vi "Update Fields Table for Spartan 5.1.vi"(8 "error in (no error)":errorcluster, 10 "Spartan Install Dir":path, 11 "Connection Refnum":T1) -> (0 "error out":errorcluster, 3 "Connection Refnum":T1)   [LabVIEW 2011]
uses:
  Summitek EXT/ODBC/SQL Controls/Connection Refnum.ctl
  Field Record.ctl
  Field DataTypes.ctl
  Field NextItem.ctl
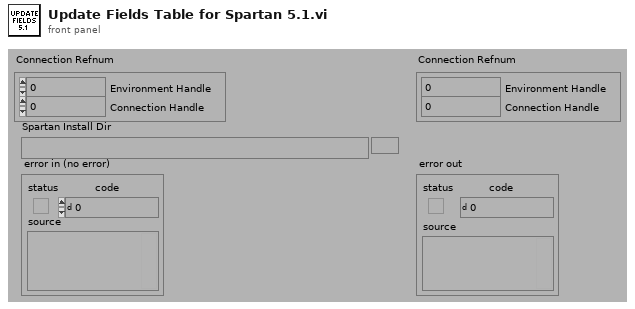
[diagram p1: front panel]
types:
  T1 = typedef "Connection Refnum.ctl" = cluster{"Environment Handle":i32, "Connection Handle":i32}
  T2 = typedef "Field Record.ctl" = cluster{"ixField":i32, "iSequenceOrder":i32, "sxFieldId":string, "sxSequenceId":string, "sDisplayName":string, "sValue":string, "sUnits":string, "nDataType":T3, "nNextItem":T4, "fSystem":bool, "fSystemValue":bool, "fRequired":bool, "fSetAtTest":bool, "fTestField":bool, "fDeleted":bool, "fIndexed":bool, "fFreeList":bool}
  T3 = typedef "Field DataTypes.ctl" = enum32{"text", "numeric", "list", "timestamp", "boolean"}
  T4 = typedef "Field NextItem.ctl" = enum32{"Reset", "Retain", "Auto-Increment"}
  T5 = enum16{"tdm_file", "tdm_channelgroup", "tdm_channel"}
  T6 = typedef "Statement Refnum.ctl" = cluster{"Statement Handle":i32, "Parameter Number":u16}
  T7 = typedef "DataFinder Indexed Property DataTypes.ctl" = enum32{"not optimized", "string", "double", "integer"}
  T8 = cluster{"DisplayName":string, "DataType":T7, "BuiltIn":bool}[]
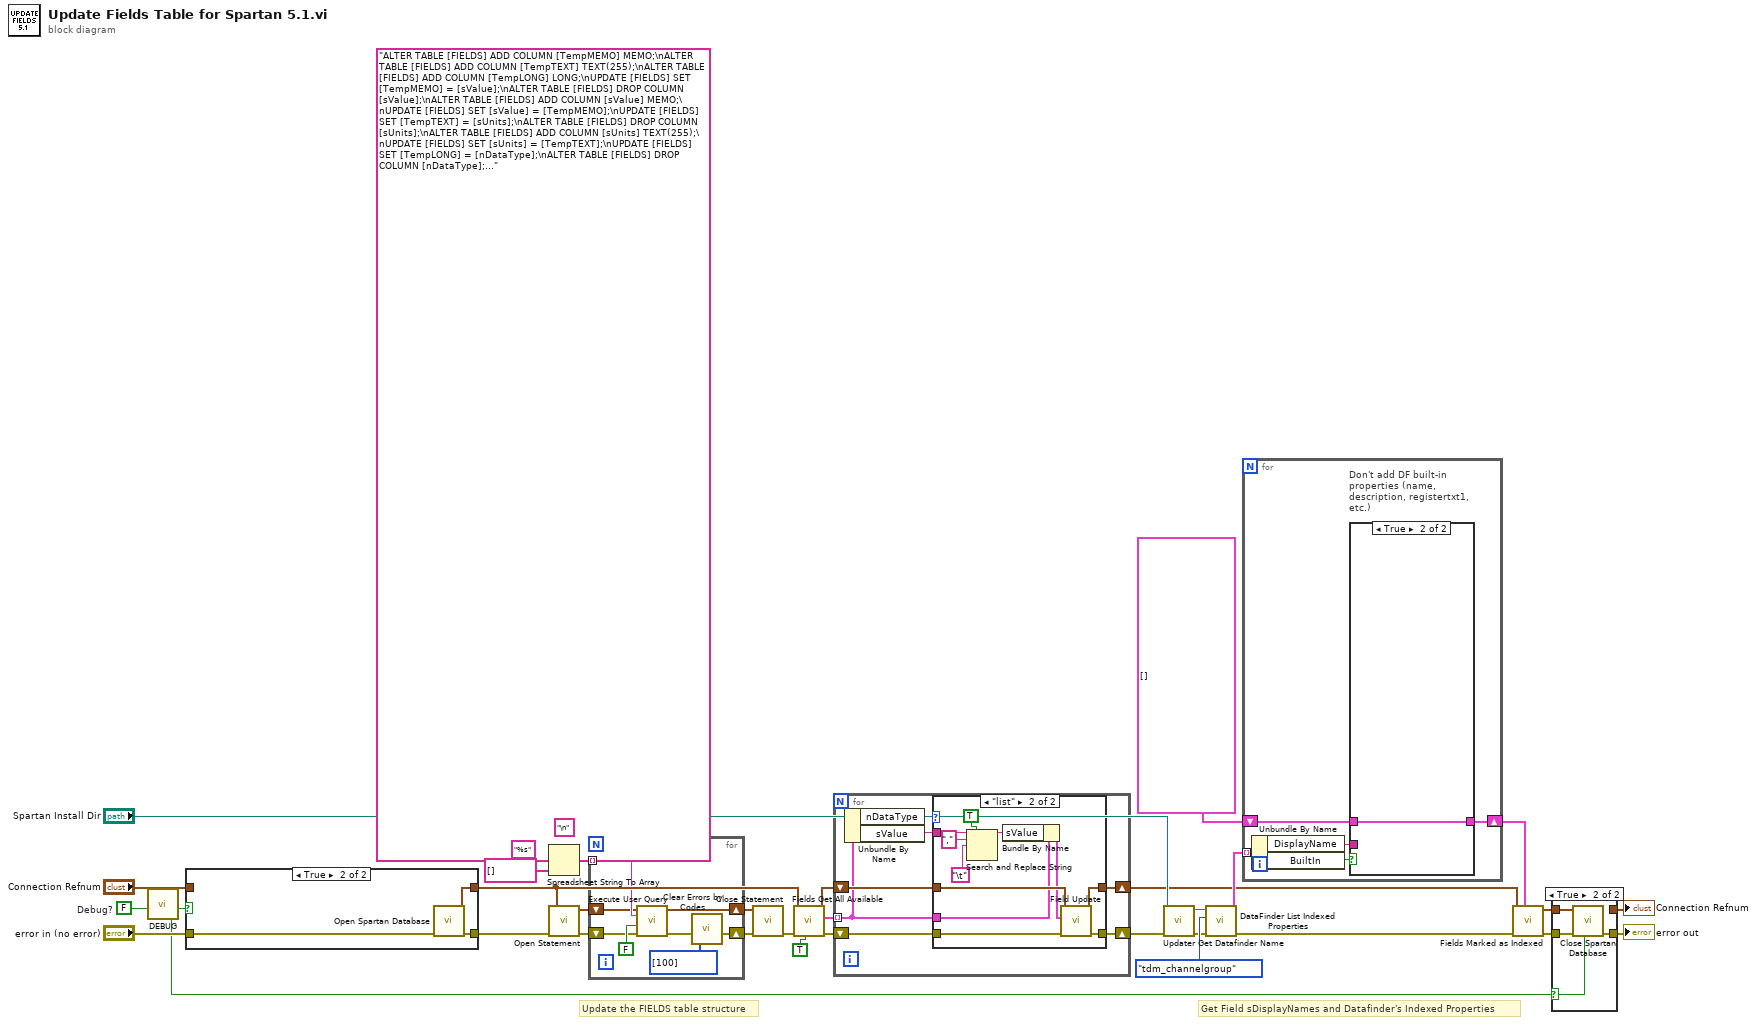
[diagram p0: block diagram]
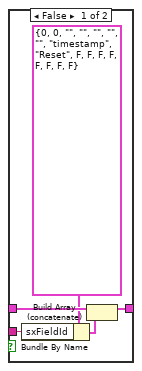
[diagram p5: hidden frame]
diagram:
  w1 = TRUE ("Combine All? (f)")
  w29 = FALSE  # Debug?
  # "Update the FIELDS table structure"
  # "Get Field sDisplayNames and Datafinder's Indexed Properties"
  n1 = call "DEBUG.vi"("Dev DEBUG? (f)"=w29) -> ("DEBUG?"=w24:bool)  [unwired: 1 in, 5 out]
  n2 = case shown="True" w24 {
    tunnel: "Connection Refnum" -> [w36 _]
    tunnel: "error in (no error)" -> [w35 w39]
    tunnel: [w35 w38] -> w9
    tunnel: [w36 w37] -> w7
    frame False {
    }
    frame True {
      n3 = call "Open Spartan Database.vi"("error in (no error)"=w39) -> ("error out"=w38:errorcluster, "Connection Refnum"=w37:T1)  [unwired: 2 in, 7 out]
    }
  }
  n4 = Spreadsheet String To Array(delimiter (Tab)="\n", format string="%s", spreadsheet string="ALTER TABLE [FIELDS] ADD COLUMN [TempMEMO] MEMO;\nALTER TABLE [FIELDS] ADD COLUMN [TempTEXT] TEXT(255);\nALTER TABLE [FIELDS] ADD COLUMN [TempLONG] LONG;\nUPDATE [FIELDS] SET [TempMEMO] = [sValue];\nALTER TABLE [FIELDS] DROP COLUMN [sValue];\nALTER TABLE [FIELDS] ADD COLUMN [sValue] MEMO;\nUPDATE [FIELDS] SET [sValue] = [TempMEMO];\nUPDATE [FIELDS] SET [TempTEXT] = [sUnits];\nALTER TABLE [FIELDS] DROP COLUMN [sUnits];\nALTER TABLE [FIELDS] ADD COLUMN [sUnits] TEXT(255);\nUPDATE [FIELDS] SET [sUnits] = [TempTEXT];\nUPDATE [FIELDS] SET [TempLONG] = [nDataType];\nALTER TABLE [FIELDS] DROP COLUMN [nDataType];\nALTER TABLE [FIELDS] ADD COLUMN [nDataType] LONG;\nUPDATE [FIELDS] SET [nDataType] = [TempLONG];\nUPDATE [FIELDS] SET [TempLONG] = [nNextItem];\nALTER TABLE [FIELDS] DROP COLUMN [nNextItem];\nALTER TABLE [FIELDS] ADD COLUMN [nNextItem] LONG;\nUPDATE [FIELDS] SET [nNextItem] = [TempLONG];\nUPDATE [FIELDS] SET [TempLONG] = [fSystem];\nALTER TABLE [FIELDS] DROP COLUMN [fSystem];\nALTER TABLE [FIELDS] ADD COLUMN [fSystem] LONG;\nUPDATE [FIELDS] SET [fSystem] = [TempLONG];\nUPDATE [FIELDS] SET [TempLONG] = [fSystemValue];\nALTER TABLE [FIELDS] DROP COLUMN [fSystemValue];\nALTER TABLE [FIELDS] ADD COLUMN [fSystemValue] LONG;\nUPDATE [FIELDS] SET [fSystemValue] = [TempLONG];\nUPDATE [FIELDS] SET [TempLONG] = [fRequired];\nALTER TABLE [FIELDS] DROP COLUMN [fRequired];\nALTER TABLE [FIELDS] ADD COLUMN [fRequired] LONG;\nUPDATE [FIELDS] SET [fRequired] = [TempLONG];\nUPDATE [FIELDS] SET [TempLONG] = [fSetAtTest];\nALTER TABLE [FIELDS] DROP COLUMN [fSetAtTest];\nALTER TABLE [FIELDS] ADD COLUMN [fSetAtTest] LONG;\nUPDATE [FIELDS] SET [fSetAtTest] = [TempLONG];\nUPDATE [FIELDS] SET [TempLONG] = [fTestField];\nALTER TABLE [FIELDS] DROP COLUMN [fTestField];\nALTER TABLE [FIELDS] ADD COLUMN [fTestField] LONG;\nUPDATE [FIELDS] SET [fTestField] = [TempLONG];\nUPDATE [FIELDS] SET [TempLONG] = [fDeleted];\nALTER TABLE [FIELDS] DROP COLUMN [fDeleted];\nALTER TABLE [FIELDS] ADD COLUMN [fDeleted] LONG;\nUPDATE [FIELDS] SET [fDeleted] = [TempLONG];\nUPDATE [FIELDS] SET [TempLONG] = [fIndexed];\nALTER TABLE [FIELDS] DROP COLUMN [fIndexed];\nALTER TABLE [FIELDS] ADD COLUMN [fIndexed] LONG;\nUPDATE [FIELDS] SET [fIndexed] = [TempLONG];\nUPDATE [FIELDS] SET [TempLONG] = [fFreeList];\nALTER TABLE [FIELDS] DROP COLUMN [fFreeList];\nALTER TABLE [FIELDS] ADD COLUMN [fFreeList] LONG;\nUPDATE [FIELDS] SET [fFreeList] = [TempLONG];\nALTER TABLE [FIELDS] DROP COLUMN [TempMEMO];\nALTER TABLE [FIELDS] DROP COLUMN [TempTEXT];\nALTER TABLE [FIELDS] DROP COLUMN [TempLONG];" ("User Query"), array type (2D Dbl)=string[] []) -> (array=w17:string[])
  n5 = call "Open Statement.vi"("error in (no error)"=w9, "Connection Refnum"=w7) -> ("error out"=w14:errorcluster, "Statement Refnum"=w13:T6)  [unwired: 4 out]
  n6 = for {
    shift-right: [w40] -> w12
    shift-left: w14 -> [w44]
    tunnel: w17 -> [w46] mode=indexing
    shift-right: [w43] -> w11
    shift-left: w13 -> [w45]
    n7 = call "Execute User Query.vi"("error in (no error)"=w44, "Return Data? (f)"=FALSE, "User Query"=w46, "Statement Refnum"=w45) -> ("error out"=w41:errorcluster, "Statement Refnum"=w43:T6)  [unwired: 2 out]
    n8 = call "Clear Errors by Codes.vi"("Error Codes\nto Clear (Empty)"=i32[] [100] ("Error Codes\nto Clear (Empty)"), "error in (no error)"=w41) -> ("error out"=w40:errorcluster)  [unwired: 5 out]
  }
  n9 = call "Close Statement.vi"("error in (no error)"=w12, "Statement Refnum"=w11) -> ("error out"=w8:errorcluster)  [unwired: 5 out]
  n10 = call "Fields Get All Available.vi"("Combine All? (f)"=w1, "Include Deleted? (F)"=w1, "error in (no error)"=w8, "Connection Refnum"=w7) -> ("error out"=w6:errorcluster, "System or ALL Combined Fields"=w2:T2[], "Connection Refnum"=w4:T1)  [unwired: 2 in, 3 out]
  n11 = for {
    shift-right: [w50] -> w5
    shift-left: w6 -> [w51]
    shift-right: [w49] -> w3
    shift-left: w4 -> [w52]
    tunnel: w2 -> [w48] mode=indexing
    n12 = Unbundle By Name(w48) -> ("nDataType"=w54:T3, "sValue"=w53:string)
    n13 = case shown="\"list\"" w54 {
      tunnel: w53 -> [_ w61]
      tunnel: w52 -> [w55 w66]
      tunnel: w51 -> [w56 w67]
      tunnel: [w56 w65] -> w50
      tunnel: [w55 w64] -> w49
      tunnel: w48 -> [_ w63]
      frame Default {
      }
      frame "list" {
        n14 = Search and Replace String(replace all?=TRUE ("replace all? (F)"), input string=w61, search string=",", replace string="\t") -> (result string=w59:string)  [unwired: 1 in, 6 out]
        n15 = Bundle By Name(cluster=w63, "sValue"=w59) -> (w62:T2)
        n16 = call "Field Update.vi"("error in (no error)"=w67, "Field Record"=w62, "Connection Refnum"=w66) -> ("error out"=w65:errorcluster, "Connection Refnum"=w64:T1)  [unwired: 7 out]
      }
    }
  }
  n17 = call "Updater Get Datafinder Name.vi"("error in (no error)"=w5, "spartan install dir"="Spartan Install Dir") -> ("error out"=w27:errorcluster, "datafinder name"=w26:string)  [unwired: 8 out]
  n18 = call "DataFinder List Indexed Properties.vi"("error in (no error)"=w27, "Type (tdm_file)"=T5."tdm_channelgroup", "DataFinder (\"My DataFinder\")"=w26) -> ("error out"=w22:errorcluster, "Indexed Properties"=w33:T8)  [unwired: 7 out]
  n19 = for {
    tunnel: w33 -> [w72] mode=indexing
    shift-right: [w68] -> w21
    shift-left: T2[] [] ("Fields In") -> [w69]
    n20 = Unbundle By Name(w72) -> ("DisplayName"=w71:string, "BuiltIn"=w70:bool)
    n21 = case "Don't add DF built-in\nproperties (name,\ndescription, registertxt1,\netc.)" shown="True" w70 {
      tunnel: w71 -> [w77 _]
      tunnel: w69 -> [w76 w78]
      tunnel: [w74 w78] -> w68
      frame False {
        n22 = Bundle By Name(cluster=T2 {"ixField"=0, "iSequenceOrder"=0, "sxFieldId"="", "sxSequenceId"="", "sDisplayName"="", "sValue"="", "sUnits"="", "nDataType"=enum."timestamp", "nNextItem"=enum."Reset", "fSystem"=FALSE, "fSystemValue"=FALSE, "fRequired"=FALSE, "fSetAtTest"=FALSE, "fTestField"=FALSE, "fDeleted"=FALSE, "fIndexed"=FALSE, "fFreeList"=FALSE} ("Field Record"), "sxFieldId"=w77) -> (w75:T2)
        n23 = Build Array (concatenate)(w76, w75) -> (w74:T2[])
      }
      frame True {
      }
    }
  }
  n24 = call "Fields Marked as Indexed.vi"("Fields In"=w21, "error in (no error)"=w22, "Connection Refnum"=w3) -> ("error out"=w19:errorcluster, "Connection Refnum"=w20:T1)  [unwired: 7 out]
  n25 = case shown="True" w24 {
    selector: w24 -> [_ w81]
    tunnel: w19 -> [w80 w84]
    tunnel: [w79 _] -> w28
    tunnel: [w80 w83] -> w30
    tunnel: w20 -> [w79 w82]
    frame False {
    }
    frame True {
      n26 = call "Close Spartan Database.vi"("Force Close? (f)"=w81, "error in (no error)"=w84, "Connection Refnum"=w82) -> ("error out"=w83:errorcluster)  [unwired: 2 in, 6 out]
    }
  }
  "Connection Refnum" <- w28
  "error out" <- w30
